vi "Area.vi"(8 "error in (no error)":errorcluster, 11 "Shape in":refnum<class "Shape.lvclass">) -> (0 "error out":errorcluster, 2 "Numeric":dbl, 3 "Shape out":refnum<class "Shape.lvclass">)   [LabVIEW 2015, in "Shape.lvclass"]
uses:
  Shape.lvclass
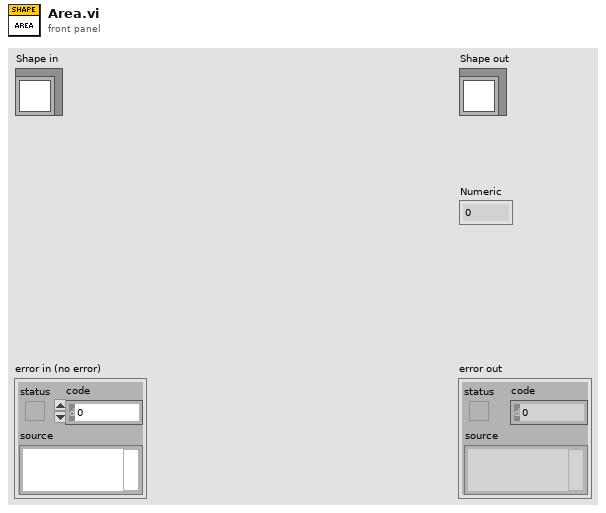
[diagram p1: front panel]
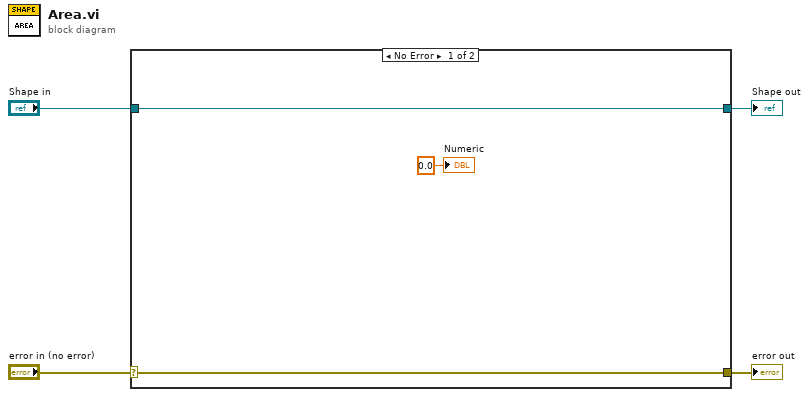
[diagram p0: block diagram]
diagram:
  n1 = case shown="No Error" "error in (no error)" {
    selector: "error in (no error)" -> [w5 w9]
    tunnel: [w5 w9] -> w3
    tunnel: [w7 w8] -> w1
    tunnel: "Shape in" -> [w7 w8]
    frame No Error {
      "Numeric" <- 0.0 ("Numeric")
    }
    frame Error {
    }
  }
  "error out" <- w3
  "Shape out" <- w1
